vi "Gradient.vi"() -> ()   [LabVIEW 2020, in "Examples.lvlib"]
uses:
  classes/Dual/Dual.lvclass/Dual.ctl
  Automatic Differentiation/Evaluate Gradient.vi/3428a883-4abf-4854-9978-3fd53a24097c.vi
  classes/Dual/Add infinitesimal to Double.vi
  classes/Dual/Read Dual Part.vi
  Automatic Differentiation/Evaluate Partial Derivative.vi/49352e5e-86b6-4795-9dd0-b0f70ab2ee45.vi
  Automatic Differentiation/Evaluate Gradient.vi/3428a883-4abf-4854-9978-3fd53a24097c.vi/5957e011-cf56-4527-b6ed-13c3a4ca997b.vi
  classes/Dual/Write a.vi
  Automatic Differentiation/Evaluate Partial Derivative.vi/49352e5e-86b6-4795-9dd0-b0f70ab2ee45.vi/5957e011-cf56-4527-b6ed-13c3a4ca997b.vi
  Tests/Multidimensional Test Function.vi
  classes/Dual/Dual.lvclass
  Examples.lvlib
  Automatic Differentiation/Automatic Differentiation.lvlib
  Tests/Tests.lvlib
panel:
  out "Gradient":dbl[](array[numeric])
  out "df(x_1,...,x_n)/dx_i":dbl
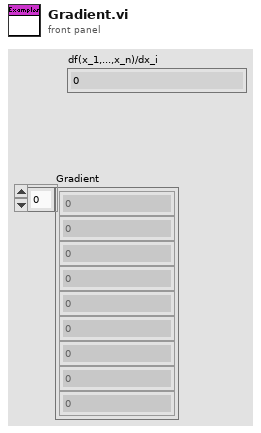
[diagram p1: front panel]
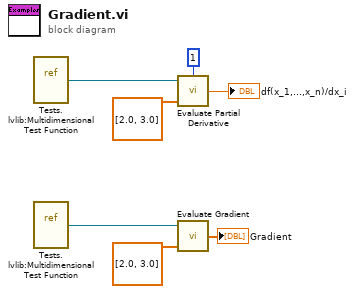
[diagram p0: block diagram]
diagram:
  n1 = vi-ref "Tests.lvlib:Multidimensional Test Function.vi"() -> (w2:refnum<vi>)
  n2 = vi-ref "Tests.lvlib:Multidimensional Test Function.vi"() -> (w1:refnum<vi>)
  n3 = call "Evaluate Partial Derivative.vi"("Partial Index"=1 ("Partial index"), "x=(x_1, ..., x_n)"=dbl[] [2.0, 3.0] ("(x_1,...,x_n)"), "Function Reference"=w2) -> ("df(x_1, ..., x_n)/dx_i"=→"df(x_1,...,x_n)/dx_i":dbl)  [unwired: 1 in]
  n4 = call "Evaluate Gradient.vi"("Point (x_1, ..., x_n)"=dbl[] [2.0, 3.0] ("(x_1,...,x_n)"), "Function Reference"=w1) -> ("Gradient"=→"Gradient":dbl[])  [unwired: 2 in]
